vi "HandleServers.vi"(8 "error in (no error)":errorcluster, 11 "S4ACS_GUI in":refnum<class "S4GUI.lvclass">) -> (0 "error out":errorcluster, 3 "S4ACS_GUI out":refnum<class "S4GUI.lvclass">)   [LabVIEW 2018, in "S4GUI.lvclass"]
uses:
  S4GUI.lvclass
  S4GUI.lvclass/S4GUI.ctl
  Acquisition/Acquisition.lvclass
  SyncBox/Sync Box.lvclass
  TCS/TCS.lvclass
  Instrument/Instrument.lvclass
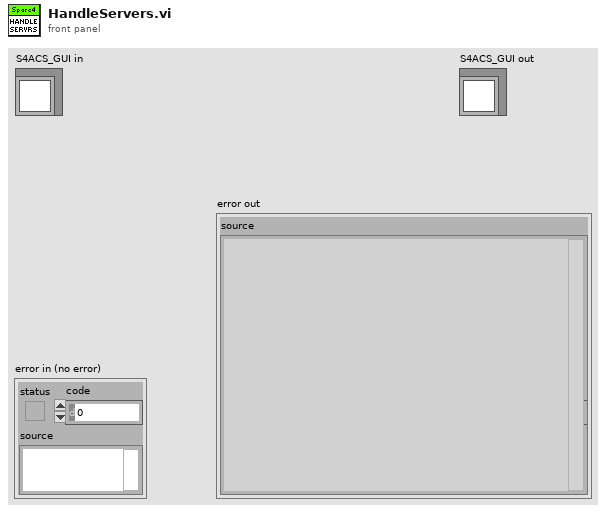
[diagram p1: front panel]
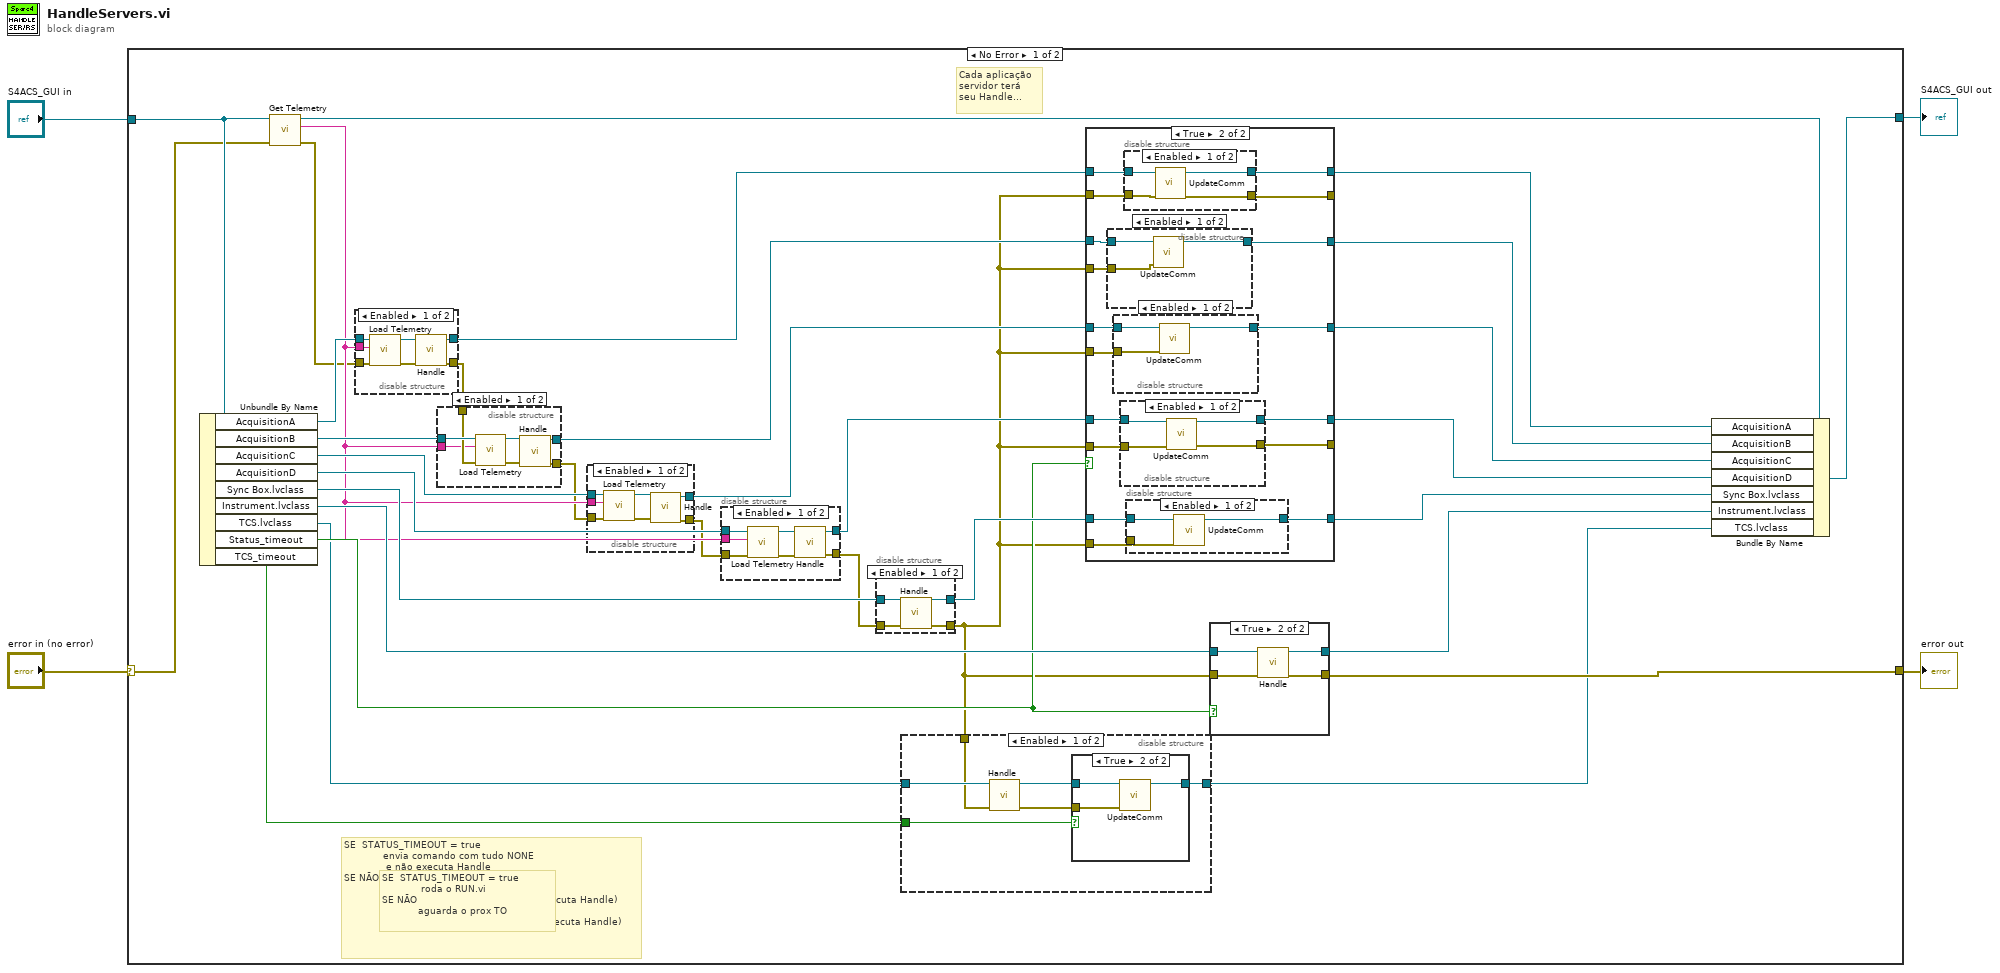
[diagram p0: block diagram]
diagram:
  n1 = case shown="No Error" "error in (no error)" {
    selector: "error in (no error)" -> [w9 w146]
    tunnel: [w34 w146] -> w3
    tunnel: [w37 w145] -> w1
    tunnel: "S4ACS_GUI in" -> [w17 w145]
    frame No Error {
      # "SE  STATUS_TIMEOUT = true\n             roda o RUN.vi\nSE NÃO\n            aguarda o prox TO"
      # "SE  STATUS_TIMEOUT = true\n             envia comando com tudo NONE\n              e não executa Handle\nSE NÃO\n             SE TODOS ESTADOS = 0\n                        Não envia comando (nao executa Handle)\n             SE NAO\n                         envia comando corrente (executa Handle)"
      # "Cada aplicação \nservidor terá \nseu Handle..."
      n2 = Unbundle By Name(w17) -> ("AcquisitionA"=w15:refnum<class "Acquisition.lvclass">, "AcquisitionB"=w14:refnum<class "Acquisition.lvclass">, "AcquisitionC"=w12:refnum<class "Acquisition.lvclass">, "AcquisitionD"=w11:refnum<class "Acquisition.lvclass">, "Sync Box.lvclass"=w36:refnum<class "Sync Box.lvclass">, "Instrument.lvclass"=w33:refnum<class "Instrument.lvclass">, "TCS.lvclass"=w19:refnum<class "TCS.lvclass">, "Status_timeout"=w21:bool, "TCS_timeout"=w7:bool)
      n3 = call-dynamic "Get Telemetry.vi"("error in (no error)"=w9, "S4ACS_GUI in"=w17) -> ("error out"=w8:errorcluster, "TCS string"=w10:string, "S4ACS_GUI out"=w16:refnum<class "S4GUI.lvclass">)  [unwired: 7 in]
      n4 = disable-structure shown="Enabled" {
        disable-tunnel: [w44 w46] -> w26
        disable-tunnel: w15 -> [w43 w46]
        disable-tunnel: [w40 w45] -> w13
        disable-tunnel: w10 -> [w39 _]
        disable-tunnel: w8 -> [w38 w45]
        frame Enabled {
          n5 = call-dynamic "Load Telemetry.vi"("error in (no error)"=w38, "TCS telemetry"=w39, "Acquisition in"=w43) -> ("error out"=w42:errorcluster, "Acquisition out"=w41:refnum<class "Acquisition.lvclass">)  [unwired: 7 in]
          n6 = call-dynamic "Handle.vi"("error in (no error)"=w42, "Acquisition in"=w41) -> ("error out"=w40:errorcluster, "Acquisition out"=w44:refnum<class "Acquisition.lvclass">)  [unwired: 8 in]
        }
        frame Disabled {
        }
      }
      n7 = disable-structure shown="Enabled" {
        disable-tunnel: [w71 w73] -> w27
        disable-tunnel: w14 -> [w70 w73]
        disable-tunnel: w13 -> [w69 w72]
        disable-tunnel: w10 -> [w68 _]
        disable-tunnel: [w65 w72] -> w6
        frame Enabled {
          n8 = call-dynamic "Load Telemetry.vi"("error in (no error)"=w69, "TCS telemetry"=w68, "Acquisition in"=w70) -> ("error out"=w66:errorcluster, "Acquisition out"=w67:refnum<class "Acquisition.lvclass">)  [unwired: 7 in]
          n9 = call-dynamic "Handle.vi"("error in (no error)"=w66, "Acquisition in"=w67) -> ("error out"=w65:errorcluster, "Acquisition out"=w71:refnum<class "Acquisition.lvclass">)  [unwired: 8 in]
        }
        frame Disabled {
        }
      }
      n10 = disable-structure shown="Enabled" {
        disable-tunnel: [w62 w64] -> w28
        disable-tunnel: w12 -> [w61 w64]
        disable-tunnel: w10 -> [w60 _]
        disable-tunnel: w6 -> [w59 w63]
        disable-tunnel: [w56 w63] -> w5
        frame Enabled {
          n11 = call-dynamic "Load Telemetry.vi"("error in (no error)"=w59, "TCS telemetry"=w60, "Acquisition in"=w61) -> ("error out"=w57:errorcluster, "Acquisition out"=w58:refnum<class "Acquisition.lvclass">)  [unwired: 7 in]
          n12 = call-dynamic "Handle.vi"("error in (no error)"=w57, "Acquisition in"=w58) -> ("error out"=w56:errorcluster, "Acquisition out"=w62:refnum<class "Acquisition.lvclass">)  [unwired: 8 in]
        }
        frame Disabled {
        }
      }
      n13 = disable-structure shown="Enabled" {
        disable-tunnel: [w53 w54] -> w35
        disable-tunnel: [w52 w55] -> w29
        disable-tunnel: w11 -> [w51 w55]
        disable-tunnel: w10 -> [w50 _]
        disable-tunnel: w5 -> [w49 w54]
        frame Enabled {
          n14 = call-dynamic "Load Telemetry.vi"("error in (no error)"=w49, "TCS telemetry"=w50, "Acquisition in"=w51) -> ("error out"=w47:errorcluster, "Acquisition out"=w48:refnum<class "Acquisition.lvclass">)  [unwired: 7 in]
          n15 = call-dynamic "Handle.vi"("error in (no error)"=w47, "Acquisition in"=w48) -> ("error out"=w53:errorcluster, "Acquisition out"=w52:refnum<class "Acquisition.lvclass">)  [unwired: 8 in]
        }
        frame Disabled {
        }
      }
      n16 = disable-structure shown="Enabled" {
        disable-tunnel: [w142 w143] -> w18
        disable-tunnel: w36 -> [w141 w144]
        disable-tunnel: [w140 w144] -> w31
        disable-tunnel: w35 -> [w139 w143]
        frame Enabled {
          n17 = call-dynamic "Handle.vi"("error in (no error)"=w139, "Sync Box in"=w141) -> ("error out"=w142:errorcluster, "Sync Box out"=w140:refnum<class "Sync Box.lvclass">)  [unwired: 8 in]
        }
        frame Disabled {
        }
      }
      n18 = disable-structure shown="Enabled" {
        disable-tunnel: w7 -> [w79 _]
        disable-tunnel: [w78 w84] -> w20
        disable-tunnel: w19 -> [w77 w84]
        disable-tunnel: w18 -> [w76 _]
        frame Enabled {
          n19 = call-dynamic "Handle.vi"("error in (no error)"=w76, "TCS in"=w77) -> ("error out"=w75:errorcluster, "TCS out"=w74:refnum<class "TCS.lvclass">)  [unwired: 8 in]
          n20 = case shown="True" w79 {
            tunnel: [w80 w83] -> w78
            tunnel: w74 -> [w80 w82]
            tunnel: w75 -> [_ w81]
            frame False {
            }
            frame True {
              n21 = call-dynamic "UpdateComm.vi"("error in (no error)"=w81, "TCS in"=w82) -> ("TCS out"=w83:refnum<class "TCS.lvclass">)  [unwired: 8 in, 1 out]
            }
          }
        }
        frame Disabled {
        }
      }
      n22 = case shown="True" w21 {
        tunnel: w31 -> [w87 w104]
        tunnel: [w87 w103] -> w30
        tunnel: w29 -> [w88 w95]
        tunnel: w28 -> [w89 w98]
        tunnel: w27 -> [w90 w101]
        tunnel: w26 -> [w91 w108]
        tunnel: w18 -> [w86 w107]
        tunnel: w18 -> [_ w100]
        tunnel: w18 -> [_ w97]
        tunnel: w18 -> [w85 w94]
        tunnel: w18 -> [_ w102]
        tunnel: [w91 w106] -> w25
        tunnel: [w90 w99] -> w24
        tunnel: [w89 w96] -> w23
        tunnel: [w88 w93] -> w22
        tunnel: [w86 w105] -> _
        tunnel: [w85 w92] -> _
        frame False {
        }
        frame True {
          n23 = disable-structure shown="Enabled" {
            disable-tunnel: w101 -> [w125 w126]
            disable-tunnel: w100 -> [w124 _]
            disable-tunnel: [w123 w126] -> w99
            frame Enabled {
              n24 = call-dynamic "UpdateComm.vi"("error in (no error)"=w124, "Acquisition in"=w125) -> ("Acquisition out"=w123:refnum<class "Acquisition.lvclass">)  [unwired: 8 in, 1 out]
            }
            frame Disabled {
            }
          }
          n25 = disable-structure shown="Enabled" {
            disable-tunnel: w98 -> [w121 w122]
            disable-tunnel: w97 -> [w120 _]
            disable-tunnel: [w119 w122] -> w96
            frame Enabled {
              n26 = call-dynamic "UpdateComm.vi"("error in (no error)"=w120, "Acquisition in"=w121) -> ("Acquisition out"=w119:refnum<class "Acquisition.lvclass">)  [unwired: 8 in, 1 out]
            }
            frame Disabled {
            }
          }
          n27 = disable-structure shown="Enabled" {
            disable-tunnel: w95 -> [w116 w118]
            disable-tunnel: w94 -> [w115 w117]
            disable-tunnel: [w114 w118] -> w93
            disable-tunnel: [w113 w117] -> w92
            frame Enabled {
              n28 = call-dynamic "UpdateComm.vi"("error in (no error)"=w115, "Acquisition in"=w116) -> ("error out"=w113:errorcluster, "Acquisition out"=w114:refnum<class "Acquisition.lvclass">)  [unwired: 8 in]
            }
            frame Disabled {
            }
          }
          n29 = disable-structure shown="Enabled" {
            disable-tunnel: w108 -> [w130 w132]
            disable-tunnel: w107 -> [w129 w131]
            disable-tunnel: [w128 w132] -> w106
            disable-tunnel: [w127 w131] -> w105
            frame Enabled {
              n30 = call-dynamic "UpdateComm.vi"("error in (no error)"=w129, "Acquisition in"=w130) -> ("error out"=w127:errorcluster, "Acquisition out"=w128:refnum<class "Acquisition.lvclass">)  [unwired: 8 in]
            }
            frame Disabled {
            }
          }
          n31 = disable-structure shown="Enabled" {
            disable-tunnel: w104 -> [w111 w112]
            disable-tunnel: [w110 w112] -> w103
            disable-tunnel: w102 -> [w109 _]
            frame Enabled {
              n32 = call-dynamic "UpdateComm.vi"("error in (no error)"=w109, "Sync Box in"=w111) -> ("Sync Box out"=w110:refnum<class "Sync Box.lvclass">)  [unwired: 8 in, 1 out]
            }
            frame Disabled {
            }
          }
        }
      }
      n33 = case shown="True" w21 {
        tunnel: [w134 w138] -> w32
        tunnel: [w133 w137] -> w34
        tunnel: w33 -> [w134 w136]
        tunnel: w18 -> [w133 w135]
        frame False {
        }
        frame True {
          n34 = call-dynamic "Handle.vi"("error in (no error)"=w135, "Instrument in"=w136) -> ("error out"=w137:errorcluster, "Instrument out"=w138:refnum<class "Instrument.lvclass">)  [unwired: 8 in]
        }
      }
      n35 = Bundle By Name(cluster=w16, "AcquisitionA"=w25, "AcquisitionB"=w24, "AcquisitionC"=w23, "AcquisitionD"=w22, "Sync Box.lvclass"=w30, "Instrument.lvclass"=w32, "TCS.lvclass"=w20) -> (w37:refnum<class "S4GUI.lvclass">)
    }
    frame Error {
    }
  }
  "error out" <- w3
  "S4ACS_GUI out" <- w1
